vi "picoTrigger.vi"(7 "Trigger Channel Settings":T1, 8 "error in (no error)":errorcluster, 9 "maxADC":i16, 10 "Trigger Settings":T2={"Trigger Enabled"=FALSE, "Trigger Source"=enum."Channel A", "Trigger Threshold (Volts)"=0.0, "Trigger Direction"=2, "Trigger Delay (samples)"=0, "Auto Trigger Time (ms)"=1000} {"Trigger Direction" items=["Rising"=2, "Falling"=3]}, 11 "Handle In":i16) -> (0 "error out":errorcluster, 1 "Range":u16, 3 "handle out":i16)   [LabVIEW 2011]
uses:
  PS2000a.dll
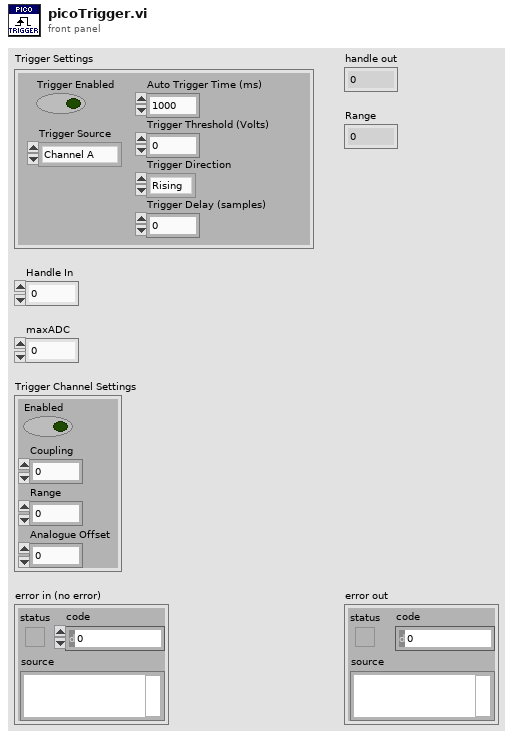
[diagram p1: front panel]
types:
  T1 = cluster{"Enabled":bool, "Coupling":i16, "Range":u16, "Analogue Offset":sgl}
  T2 = cluster{"Trigger Enabled":bool, "Trigger Source":enum16{"Channel A", "Channel B", "Channel C", "Channel D", "Ext."}, "Trigger Threshold (Volts)":dbl, "Trigger Direction":u16, "Trigger Delay (samples)":u32, "Auto Trigger Time (ms)":i16}
  T3 = enum16{"Channel A", "Channel B", "Channel C", "Channel D", "Ext."}
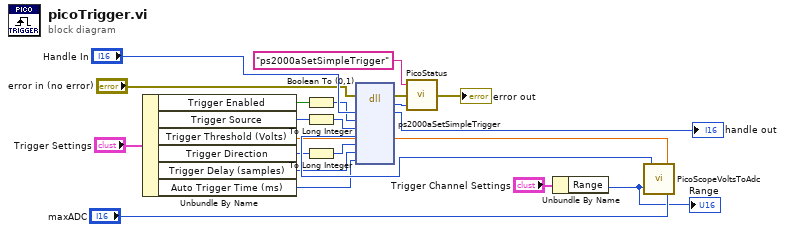
[diagram p0: block diagram]
diagram:
  n1 = Unbundle By Name("Trigger Settings") -> ("Trigger Enabled"=w8:bool, "Trigger Source"=w9:T3, "Trigger Threshold (Volts)"=w14:dbl, "Trigger Direction"=w10:u16, "Trigger Delay (samples)"=w11:u32, "Auto Trigger Time (ms)"=w12:i16)
  n2 = Boolean To (0,1)(Boolean=w8) -> (0, 1=w4:i16)
  n3 = To Long Integer(number=w9) -> (32bit integer=w1:i32)
  n4 = To Long Integer(number=w10) -> (32bit integer=w2:i32)
  n5 = Unbundle By Name("Trigger Channel Settings") -> ("Range"=w20:u16)
  "Range" <- w20
  n6 = call "PicoScopeVoltsToAdc.vi"("Max_adc"="maxADC", "Volts"=w14, "Range Index"=w20) -> ("ADC count"=w15:i16)
  n7 = dll-call lib="ps2000a.dll" fn="ps2000aSetSimpleTrigger" ("ps2000a.dll:_ps3000_open_unit@0")(error in="error in (no error)", "handle"="Handle In", "enabled"=w4, "source"=w1, "threshold"=w15, "direction"=w2, "delay"=w11, "autoTrigger_ms"=w12) -> (error out=w6:errorcluster, "PICO_STATUS"=w5:u32, "handle"=→"handle out":i16)  [unwired: 8 in, 1 out]
  n8 = call "PicoStatus.vi"("PICO STATUS"=w5, "error in"=w6, "source"="ps2000aSetSimpleTrigger") -> ("error out"=→"error out":errorcluster)
